vi "SWERVE_DRIVE_DASH_WRITE.vi"   [LabVIEW 2019]
uses:
  SWERVE_DRIVE_GLOBALS.vi
  <vilib>/Rock Robotics/Network Tables/NT Write Numeric Array.vi
  <vilib>/Rock Robotics/Network Tables/NT Write Boolean Array.vi
  <vilib>/Rock Robotics/Network Tables/NT Write Boolean.vi
  <vilib>/Rock Robotics/Network Tables/NT Write Number.vi
  <vilib>/Rock Robotics/WPI/ThirdParty/JAS_Junk/TrajLib/Trajectory_Library.lvlib
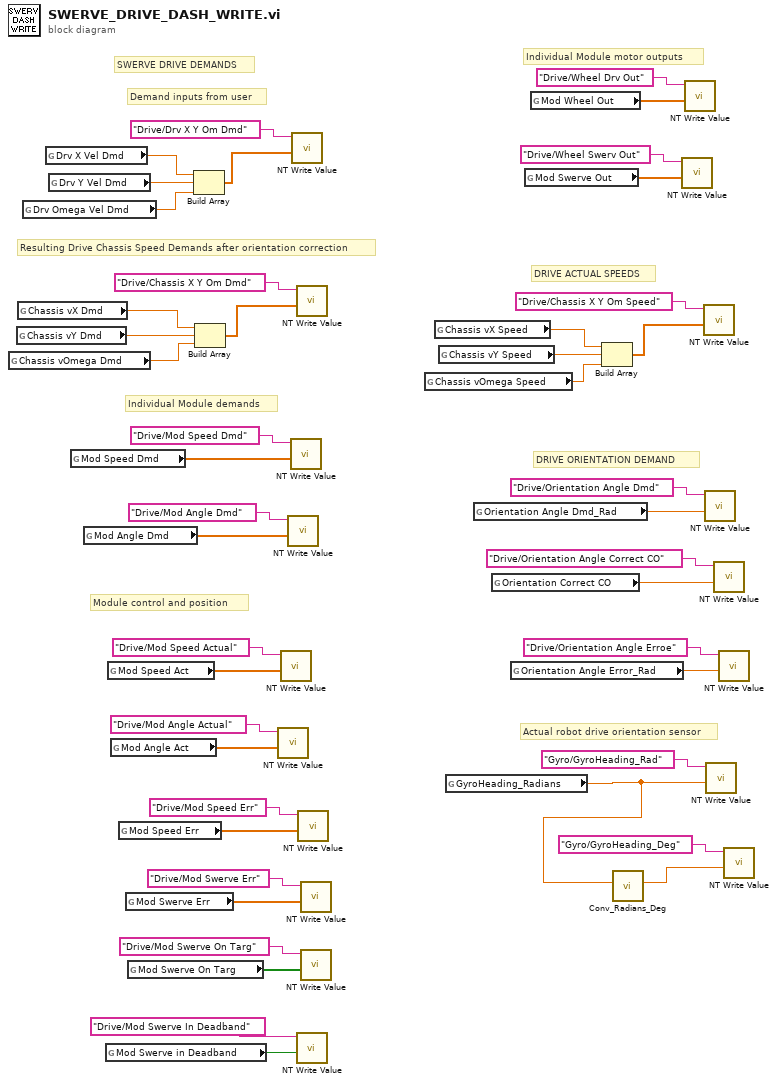
[diagram p0: block diagram]
diagram:
  # "Module control and position"
  # "Actual robot drive orientation sensor"
  # "DRIVE ACTUAL SPEEDS"
  # "DRIVE ORIENTATION DEMAND"
  # "Individual Module motor outputs"
  # "Individual Module demands"
  # "Resulting Drive Chassis Speed Demands after orientation correction"
  # "Demand inputs from user"
  # "SWERVE DRIVE DEMANDS"
  n1 = global read "SWERVE_DRIVE_GLOBALS.vi" "Chassis vOmega Dmd"() -> (w20:dbl)
  n2 = global read "SWERVE_DRIVE_GLOBALS.vi" "Chassis vY Dmd"() -> (w21:dbl)
  n3 = global read "SWERVE_DRIVE_GLOBALS.vi" "Chassis vX Dmd"() -> (w22:dbl)
  n4 = global read "SWERVE_DRIVE_GLOBALS.vi" "Drv Omega Vel Dmd"() -> (w23:dbl)
  n5 = global read "SWERVE_DRIVE_GLOBALS.vi" "Drv X Vel Dmd"() -> (w25:dbl)
  n6 = global read "SWERVE_DRIVE_GLOBALS.vi" "Drv Y Vel Dmd"() -> (w24:dbl)
  n7 = global read "SWERVE_DRIVE_GLOBALS.vi" "Mod Speed Dmd"() -> (w19:dbl[])
  n8 = global read "SWERVE_DRIVE_GLOBALS.vi" "Mod Angle Dmd"() -> (w18:dbl[])
  n9 = global read "SWERVE_DRIVE_GLOBALS.vi" "Mod Swerve in Deadband"() -> (w13:bool)
  n10 = global read "SWERVE_DRIVE_GLOBALS.vi" "Mod Speed Act"() -> (w17:dbl[])
  n11 = global read "SWERVE_DRIVE_GLOBALS.vi" "Mod Angle Act"() -> (w16:dbl[])
  n12 = global read "SWERVE_DRIVE_GLOBALS.vi" "Mod Speed Err"() -> (w15:dbl[])
  n13 = global read "SWERVE_DRIVE_GLOBALS.vi" "Mod Swerve Err"() -> (w14:dbl[])
  n14 = global read "SWERVE_DRIVE_GLOBALS.vi" "Mod Swerve On Targ"() -> (w12:bool[])
  n15 = Build Array(w25, w24, w23) -> (w29:dbl[])
  n16 = Build Array(w22, w21, w20) -> (w31:dbl[])
  n17 = call-poly <vilib>:"NT Write Value.vi"("Numeric Array"=w16, "Name"="Drive/Mod Angle Actual") -> ()  [unwired: 9 in, 1 out]
  n18 = call-poly <vilib>:"NT Write Value.vi"("Numeric Array"=w17, "Name"="Drive/Mod Speed Actual") -> ()  [unwired: 9 in, 1 out]
  n19 = call-poly <vilib>:"NT Write Value.vi"("Numeric Array"=w18, "Name"="Drive/Mod Angle Dmd") -> ()  [unwired: 9 in, 1 out]
  n20 = call-poly <vilib>:"NT Write Value.vi"("Numeric Array"=w19, "Name"="Drive/Mod Speed Dmd") -> ()  [unwired: 9 in, 1 out]
  n21 = call-poly <vilib>:"NT Write Value.vi"("Numeric Array"=w29, "Name"="Drive/Drv X Y Om Dmd") -> ()  [unwired: 9 in, 1 out]
  n22 = call-poly <vilib>:"NT Write Value.vi"("Numeric Array"=w31, "Name"="Drive/Chassis X Y Om Dmd") -> ()  [unwired: 9 in, 1 out]
  n23 = call-poly <vilib>:"NT Write Value.vi"("Boolean"=w13, "Name"="Drive/Mod Swerve In Deadband") -> ()  [unwired: 9 in, 1 out]
  n24 = call-poly <vilib>:"NT Write Value.vi"("Numeric Array"=w15, "Name"="Drive/Mod Speed Err") -> ()  [unwired: 9 in, 1 out]
  n25 = call-poly <vilib>:"NT Write Value.vi"("Numeric Array"=w14, "Name"="Drive/Mod Swerve Err") -> ()  [unwired: 9 in, 1 out]
  n26 = call-poly <vilib>:"NT Write Value.vi"("Boolean Array"=w12, "Name"="Drive/Mod Swerve On Targ") -> ()  [unwired: 9 in, 1 out]
  n27 = global read "SWERVE_DRIVE_GLOBALS.vi" "Chassis vOmega Speed"() -> (w1:dbl)
  n28 = global read "SWERVE_DRIVE_GLOBALS.vi" "Chassis vX Speed"() -> (w3:dbl)
  n29 = global read "SWERVE_DRIVE_GLOBALS.vi" "Chassis vY Speed"() -> (w2:dbl)
  n30 = global read "SWERVE_DRIVE_GLOBALS.vi" "GyroHeading_Radians"() -> (w4:dbl)
  n31 = global read "SWERVE_DRIVE_GLOBALS.vi" "Orientation Angle Dmd_Rad"() -> (w9:dbl)
  n32 = global read "SWERVE_DRIVE_GLOBALS.vi" "Orientation Correct CO"() -> (w8:dbl)
  n33 = global read "SWERVE_DRIVE_GLOBALS.vi" "Orientation Angle Error_Rad"() -> (w7:dbl)
  n34 = global read "SWERVE_DRIVE_GLOBALS.vi" "Mod Swerve Out"() -> (w11:dbl[])
  n35 = global read "SWERVE_DRIVE_GLOBALS.vi" "Mod Wheel Out"() -> (w10:dbl[])
  n36 = Build Array(w3, w2, w1) -> (w39:dbl[])
  n37 = call <vilib>:"Conv_Radians_Deg.vi"("Radians"=w4) -> ("Degrees"=w5:dbl)  [unwired: 10 in]
  n38 = call-poly <vilib>:"NT Write Value.vi"("Numeric Array"=w11, "Name"="Drive/Wheel Swerv Out") -> ()  [unwired: 9 in, 1 out]
  n39 = call-poly <vilib>:"NT Write Value.vi"("Numeric Array"=w10, "Name"="Drive/Wheel Drv Out") -> ()  [unwired: 9 in, 1 out]
  n40 = call-poly <vilib>:"NT Write Value.vi"("Numeric Array"=w39, "Name"="Drive/Chassis X Y Om Speed") -> ()  [unwired: 9 in, 1 out]
  n41 = call-poly <vilib>:"NT Write Value.vi"("Numeric"=w9, "Name"="Drive/Orientation Angle Dmd") -> ()  [unwired: 9 in, 1 out]
  n42 = call-poly <vilib>:"NT Write Value.vi"("Numeric"=w4, "Name"="Gyro/GyroHeading_Rad") -> ()  [unwired: 9 in, 1 out]
  n43 = call-poly <vilib>:"NT Write Value.vi"("Numeric"=w8, "Name"="Drive/Orientation Angle Correct CO") -> ()  [unwired: 9 in, 1 out]
  n44 = call-poly <vilib>:"NT Write Value.vi"("Numeric"=w7, "Name"="Drive/Orientation Angle Erroe") -> ()  [unwired: 9 in, 1 out]
  n45 = call-poly <vilib>:"NT Write Value.vi"("Numeric"=w5, "Name"="Gyro/GyroHeading_Deg") -> ()  [unwired: 9 in, 1 out]
